vi "RDS Serial Handle Frame.vi"(8 "error in (no error)":errorcluster, 10 "RDS Serial Frame":refnum<class "RDS Serial Frame.lvclass">, 11 "LSR Instrument in":refnum<class "LSR Instrument.lvclass">) -> (0 "error out":errorcluster, 3 "LSR Instrument out":refnum<class "LSR Instrument.lvclass">)   [LabVIEW 2015, in "LSR Instrument.lvlib" / "LSR Instrument.lvclass"]
uses:
  LSR Instrument.lvclass
  Libraries/RDS Serial Handler/RDS Serial Frame.lvclass
  Actors/RDS Parent Actor/RDS Parent Actor/RDS Parent Actor.lvclass
  LSR Transmission/LSR Transmission.lvlib
  Libraries/RDS Framework/RDS Message Class/RDS Message.lvclass
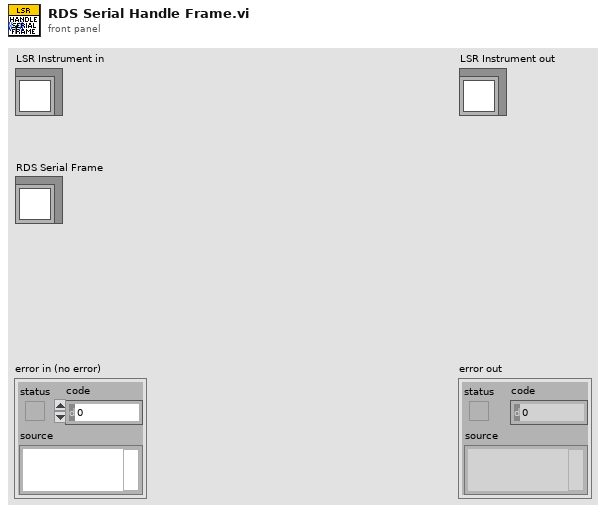
[diagram p1: front panel]
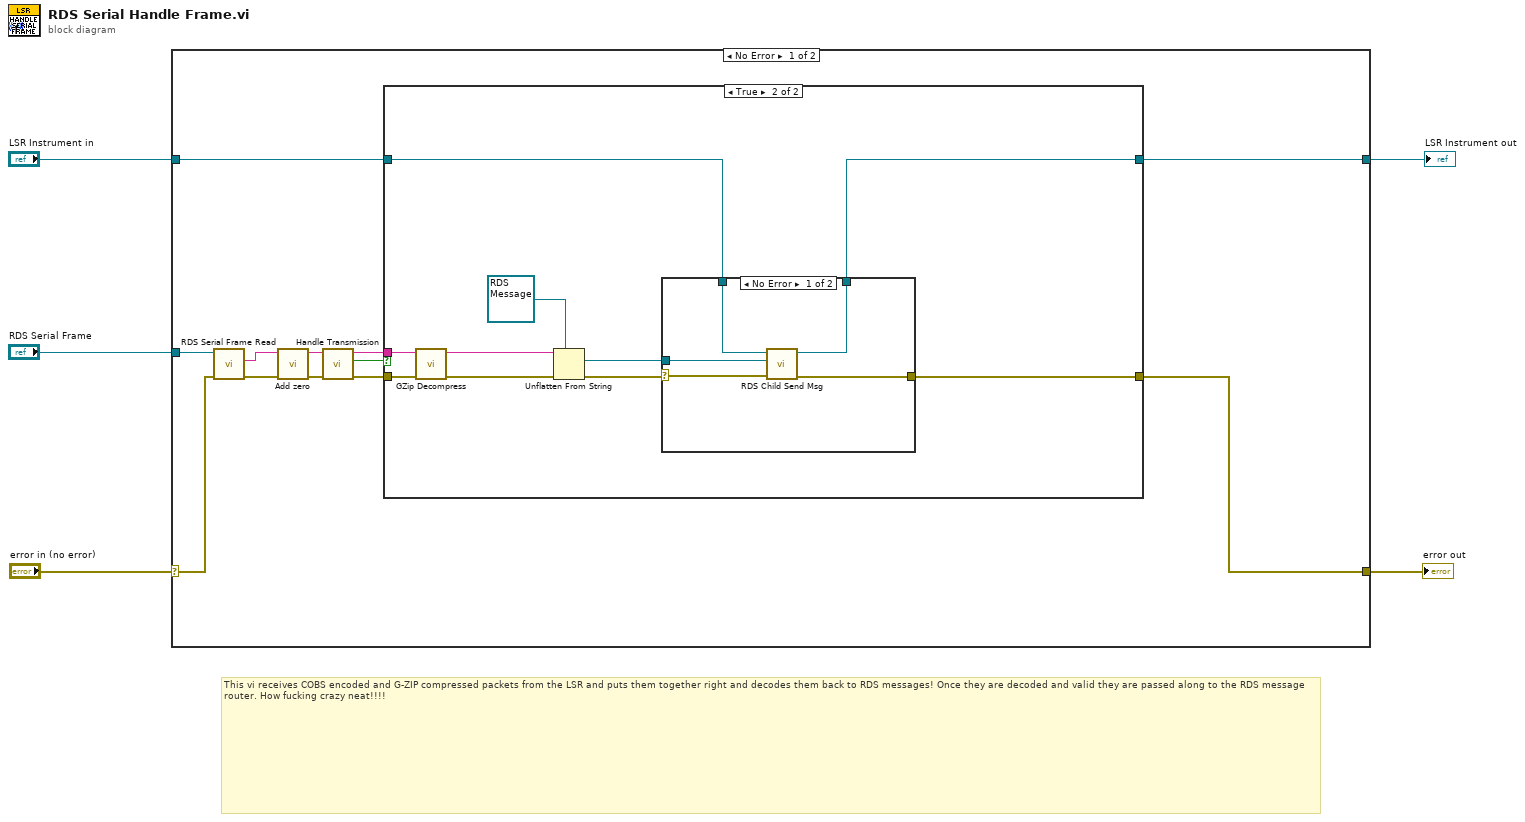
[diagram p0: block diagram]
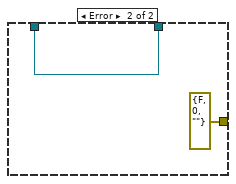
[diagram p3: hidden frame]
diagram:
  # "This vi receives COBS encoded and G-ZIP compressed packets from the LSR and puts them together right and decodes them back to RDS messages! Once they are decoded and valid they are passed along to the RDS message router. How fucking crazy neat!!!!"
  n1 = case shown="No Error" "error in (no error)" {
    selector: "error in (no error)" -> [w9 w37]
    tunnel: "RDS Serial Frame" -> [w17 _]
    tunnel: "LSR Instrument in" -> [w8 w38]
    tunnel: [w7 w38] -> w2
    tunnel: [w6 w37] -> w1
    frame No Error {
      n2 = call "RDS Serial Frame Read.vi"("error in (no error)"=w9, "RDS Serial Frame in"=w17) -> ("error out"=w10:errorcluster, "Serial String"=w11:string)  [unwired: 6 in, 2 out]
      n3 = call "Add zero.vi"("error in (no error)"=w10, "String in"=w11) -> ("error out"=w12:errorcluster, "String out"=w13:string)  [unwired: 8 in]
      n4 = call "Handle Transmission.vi"("error in (no error)"=w12, "Stuffed Data"=w13) -> ("error out"=w15:errorcluster, "Transmission valid?"=w14:bool, "Transmission"=w16:string)  [unwired: 7 in]
      n5 = case shown="True" w14 {
        tunnel: w16 -> [_ w29]
        tunnel: w15 -> [w18 w28]
        tunnel: w8 -> [w19 w24]
        tunnel: [w19 w23] -> w7
        tunnel: [w18 w20] -> w6
        frame False {
        }
        frame True {
          n6 = call "GZip Decompress.vi"("error in (no error)"=w28, "GZip compressed string"=w29) -> ("error out"=w21:errorcluster, "Decompressed string"=w26:string)  [unwired: 8 in]
          n7 = Unflatten From String(type=refnum<class "RDS Message.lvclass"> refnum ("RDS Child Messages.lvlib:RDS Message.lvclass"), binary string=w26, error in (no error)=w21) -> (value=w25:refnum<class "RDS Message.lvclass">, error out=w22:errorcluster)  [unwired: 2 in, 1 out]
          n8 = case shown="No Error" w22 {
            selector: w22 -> [w31 _]
            tunnel: w25 -> [w34 _]
            tunnel: w24 -> [w33 w36]
            tunnel: [w32 w36] -> w23
            tunnel: [w30 errorcluster {"status"=FALSE, "code"=0, "source"=""} ("error out")] -> w20
            frame No Error {
              n9 = call "RDS Child Send Msg.vi"("error in (no error)"=w31, "RDS Message"=w34, "RDS Parent Actor in"=w33) -> ("error out"=w30:errorcluster, "RDS Parent Actor out"=w32:refnum<class "LSR Instrument.lvclass">)  [unwired: 7 in]
            }
            frame Error {
            }
          }
        }
      }
    }
    frame Error {
    }
  }
  "error out" <- w1
  "LSR Instrument out" <- w2
